vi "amc_Format XML.vi"(8 "error in (no error)":errorcluster, 11 "Message":T1={"Name"="cRIO", "Value"="controlSM", "Attributes"={"keys"=[], "values"=[]}, "Receiver Host"="MachinePg", "Receiver Process"="", "Source Host"="", "Source Process"="", "Priority Message"=FALSE, "Acknowledge Message"=FALSE}) -> (0 "error out":errorcluster, 3 "Message XML String":string)   [LabVIEW 2012, in "REx_Springboard.lvlib" / "TLB_Dependencies.lvlib"]
uses:
  TLB_Dependencies.lvlib
  amc_Message.ctl
  <vilib>/FTP/util/Keyed Array.ctl
  <vilib>/FTP/NI_FTP.lvlib
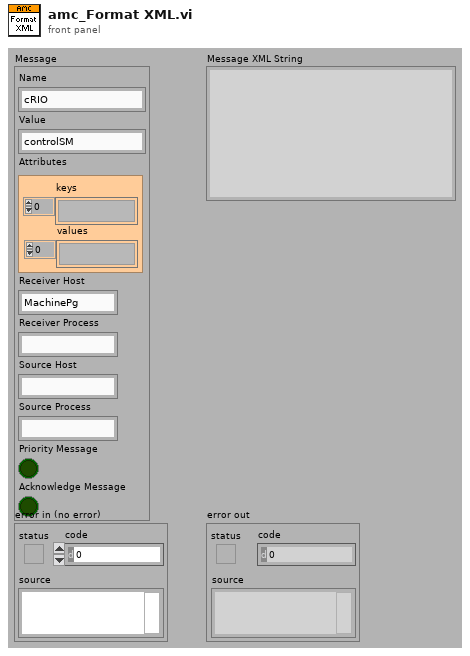
[diagram p1: front panel]
types:
  T1 = typedef "REx_Springboard.lvlib/TLB_Dependencies.lvlib/amc_Message.ctl" = cluster{"Name":string, "Value":string, "Attributes":T2, "Receiver Host":string, "Receiver Process":string, "Source Host":string, "Source Process":string, "Priority Message":bool, "Acknowledge Message":bool}
  T2 = typedef "NI_FTP.lvlib/Keyed Array.ctl" = cluster{"keys":string[], "values":string[]}
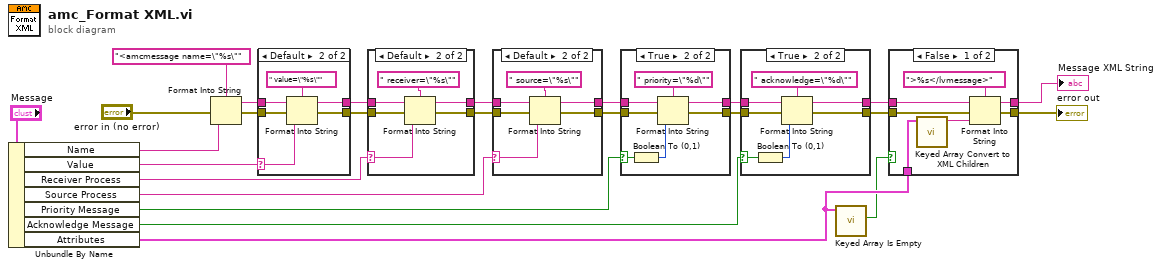
[diagram p0: block diagram]
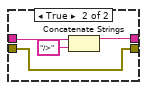
[diagram p4: hidden frame]
diagram:
  n1 = Unbundle By Name("Message") -> ("Name"=w21:string, "Value"=w22:string, "Receiver Process"=w23:string, "Source Process"=w24:string, "Priority Message"=w7:bool, "Acknowledge Message"=w4:bool, "Attributes"=w25:T2)
  n2 = Format Into String(format string="<amcmessage name=\"%s\"", error in="error in (no error)", w21) -> (resulting string=w16:string, error out=w13:errorcluster)  [unwired: 1 in]
  n3 = case shown="Default" w22 {
    selector: w22 -> [_ w31]
    tunnel: w16 -> [w27 w33]
    tunnel: [w27 w30] -> w17
    tunnel: w13 -> [w26 w29]
    tunnel: [w26 w28] -> w12
    frame "" {
    }
    frame Default {
      n4 = Format Into String(format string=" value=\"%s\"", initial string=w33, error in=w29, w31) -> (resulting string=w30:string, error out=w28:errorcluster)
    }
  }
  n5 = case shown="Default" w23 {
    selector: w23 -> [_ w39]
    tunnel: w17 -> [w35 w41]
    tunnel: [w35 w38] -> w18
    tunnel: w12 -> [w34 w37]
    tunnel: [w34 w36] -> w11
    frame "" {
    }
    frame Default {
      n6 = Format Into String(format string=" receiver=\"%s\"", initial string=w41, error in=w37, w39) -> (resulting string=w38:string, error out=w36:errorcluster)
    }
  }
  n7 = case shown="Default" w24 {
    selector: w24 -> [_ w47]
    tunnel: w18 -> [w43 w49]
    tunnel: [w43 w46] -> w8
    tunnel: w11 -> [w42 w45]
    tunnel: [w42 w44] -> w6
    frame "" {
    }
    frame Default {
      n8 = Format Into String(format string=" source=\"%s\"", initial string=w49, error in=w45, w47) -> (resulting string=w46:string, error out=w44:errorcluster)
    }
  }
  n9 = case shown="True" w7 {
    selector: w7 -> [_ w53]
    tunnel: w8 -> [w51 w58]
    tunnel: [w51 w56] -> w5
    tunnel: w6 -> [w50 w55]
    tunnel: [w50 w54] -> w3
    frame False {
    }
    frame True {
      n10 = Boolean To (0,1)(Boolean=w53) -> (0, 1=w52:i16)
      n11 = Format Into String(format string=" priority=\"%d\"", initial string=w58, error in=w55, w52) -> (resulting string=w56:string, error out=w54:errorcluster)
    }
  }
  n12 = case shown="True" w4 {
    selector: w4 -> [_ w62]
    tunnel: w5 -> [w60 w67]
    tunnel: [w60 w65] -> w2
    tunnel: w3 -> [w59 w64]
    tunnel: [w59 w63] -> w1
    frame False {
    }
    frame True {
      n13 = Boolean To (0,1)(Boolean=w62) -> (0, 1=w61:i16)
      n14 = Format Into String(format string=" acknowledge=\"%d\"", initial string=w67, error in=w64, w61) -> (resulting string=w65:string, error out=w63:errorcluster)
    }
  }
  n15 = call "Keyed Array Is Empty.vi"("array in"=w25) -> ("empty?"=w19:bool)  [unwired: 6 out]
  n16 = case shown="False" w19 {
    tunnel: w2 -> [w74 w77]
    tunnel: [w73 w78] -> w9
    tunnel: w25 -> [w72 _]
    tunnel: w1 -> [w69 w75]
    tunnel: [w68 w75] -> w10
    frame False {
      n17 = call "Keyed Array Convert to XML Children.vi"("Keyed Array"=w72) -> ("KA XML Children"=w70:string)  [unwired: 10 out]
      n18 = Format Into String(format string=">%s</lvmessage>", initial string=w74, error in=w69, w70) -> (resulting string=w73:string, error out=w68:errorcluster)
    }
    frame True {
      n19 = Concatenate Strings(w77, "/>" ("string")) -> (w78:string)
    }
  }
  "Message XML String" <- w9
  "error out" <- w10
